vi "Get configuration chain.vi"(8 "error in (no error)":errorcluster, 11 "RSABase in":refnum<class "RSA.lvclass">) -> (0 "error out":errorcluster, 1 "class name":string[](array[string]), 2 "configuration chain":variant[](array[variant]), 3 "RSABase out":refnum<class "RSA.lvclass">)   [LabVIEW 2012, in "RSA.lvclass"]
doc: "Returns an array of variants containing the configuration clusters of each class in the inheritance chain (lowest child class first), together with an array of all class names in the inheritance chain.\n\nFor classes without configuration cluster, the configuration chain contains empty variants."
uses:
  RSA.lvclass
  <vilib>/Distrio/Murmex/Murmex/Murmex.lvclass
  RSA.lvclass/RSA.ctl
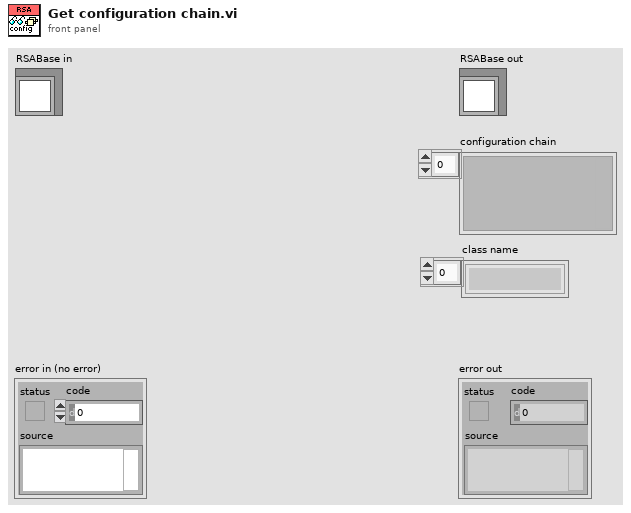
[diagram p1: front panel]
types:
  T1 = typedef "RSA.lvclass/configurationcluster.ctl" = cluster{"initialised array":dbl[]}
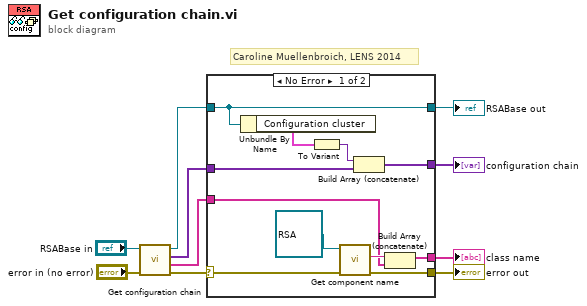
[diagram p0: block diagram]
diagram:
  # "Caroline Muellenbroich, LENS 2014"
  n1 = call-parent "Get configuration chain.vi"("error in (no error)"="error in (no error)", "MurmexBase in"="RSABase in") -> ("error out"=w8:errorcluster, "class name"=w5:string[], "configuration chain"=w4:variant[], "MurmexBase out"=w3:refnum<class "RSA.lvclass">)  [unwired: 6 in]
  n2 = case shown="No Error" w8 {
    selector: w8 -> [w21 w25]
    tunnel: [w18 w22] -> w7
    tunnel: [w17 w25] -> w6
    tunnel: w5 -> [w16 w22]
    tunnel: w4 -> [w14 w23]
    tunnel: w3 -> [w11 w24]
    tunnel: [w11 w24] -> w2
    tunnel: [w12 w23] -> w1
    frame No Error {
      n3 = Unbundle By Name(w11) -> ("Configuration cluster"=w13:T1)
      n4 = To Variant(anything=w13) -> (Variant=w15:variant)
      n5 = call <vilib>:"Get component name.vi"("error in (no error)"=w21, "Murmex in"=refnum<class "RSA.lvclass"> refnum ("RSA")) -> ("error out"=w17:errorcluster, "component name"=w19:string)  [unwired: 7 in, 1 out]
      n6 = Build Array (concatenate)(w15, w14) -> (w12:variant[])
      n7 = Build Array (concatenate)(w19, w16) -> (w18:string[])
    }
    frame Error {
    }
  }
  "error out" <- w6
  "RSABase out" <- w2
  "configuration chain" <- w1
  "class name" <- w7
